vi "e.gate ASCII Write Value - Boolean.vi"(6 "Value":bool, 8 "error in (no error)":errorcluster, 9 "Channel":i32, 11 "e.gate Configuration In":T1) -> (0 "error out":errorcluster, 3 "connection ID Out":T1)   [LabVIEW 2016]
doc: "<B>AMC - Analytik & Messtechnik GmbH Chemnitz</B>\n\nLabVIEW Drivers for e.gate / e.pac series from Gantner Instruments\n\nThis VI writes a value specified by <B>Channel</B> to a device specified by <B>connection ID In</B>."
uses:
  e.gate Configuration.ctl
  e.gate Channel Data.ctl
  e.gate Data Type.ctl
  e.gate Protocol Type.ctl
  e.gate Module  Data.ctl
  e.gateHSP_DLLhandle.ctl
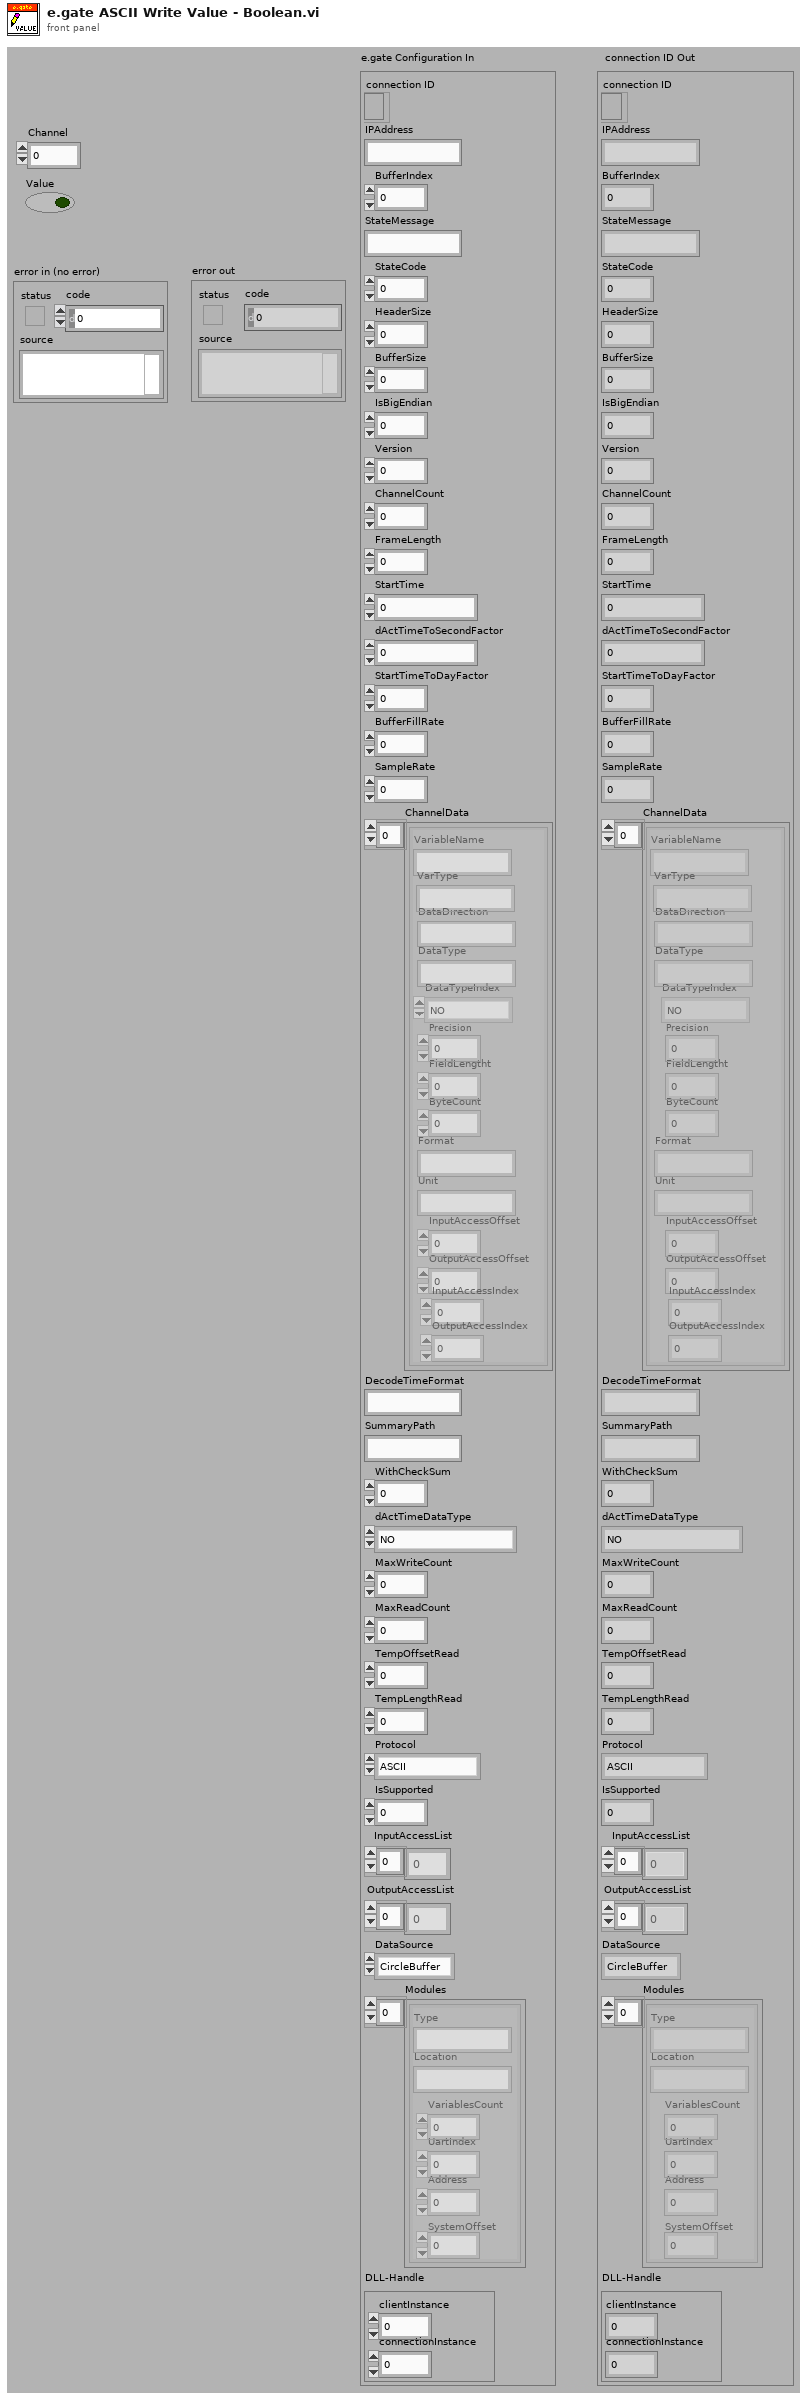
[diagram p1: front panel]
types:
  T1 = typedef "e.gate Configuration.ctl" = cluster{"connection ID":refnum<k5>, "IPAddress":string, "BufferIndex":i32, "StateMessage":string, "StateCode":i8, "HeaderSize":i32, "BufferSize":i32, "IsBigEndian":i32, "Version":i32, "ChannelCount":i32, "FrameLength":i32, "StartTime":dbl, "dActTimeToSecondFactor":dbl, "StartTimeToDayFactor":dbl, "BufferFillRate":dbl, "SampleRate":dbl, "ChannelData":T2[], "DecodeTimeFormat":string, "SummaryPath":string, "WithCheckSum":i32, "dActTimeDataType":T3, "MaxWriteCount":i32, "MaxReadCount":i32, "TempOffsetRead":i32, "TempLengthRead":i32, "Protocol":T4, "IsSupported":i32, "InputAccessList":i32[], "OutputAccessList":i32[], "DataSource":enum16{"CircleBuffer", "test.con Logger", "test.con Archive"}, "Modules":T5[], "DLL-Handle":T6}
  T2 = typedef "e.gate Channel Data.ctl" = cluster{"VariableName":string, "DataDirection":string, "DataType":string, "DataTypeIndex":T3, "Precision":i16, "FieldLengtht":i16, "ByteCount":i32, "Format":string, "Unit":string, "InputAccessOffset":i32, "OutputAccessOffset":i16, "InputAccessIndex":i16, "OutputAccessIndex":i16, "VarType":string}
  T3 = typedef "e.gate Data Type.ctl" = enum16{"NO", "BOOL", "SINT8", "USINT8", "SINT16", "USINT16", "SINT32", "USINT32", "FLOAT", "SET8", "SET16", "SET32", "DOUBLE", "SINT64", "USINT64", "SET64"}
  T4 = typedef "e.gate Protocol Type.ctl" = enum16{"ASCII", "HighspeedPort Online", "HighspeedPort Buffer", "eGateHighspeedPortDLL "}
  T5 = typedef "e.gate Module  Data.ctl" = cluster{"Type":string, "Location":string, "VariablesCount":i16, "UartIndex":i16, "Address":i16, "SystemOffset":i16}
  T6 = typedef "e.gateHSP_DLLhandle.ctl" = cluster{"clientInstance":i32, "connectionInstance":i32}
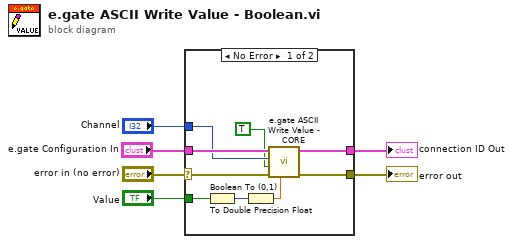
[diagram p0: block diagram]
diagram:
  n1 = case shown="No Error" "error in (no error)" {
    selector: "error in (no error)" -> [w15 w17]
    tunnel: "e.gate Configuration In" -> [w14 w16]
    tunnel: "Channel" -> [w8 _]
    tunnel: [w13 w16] -> w3
    tunnel: [w12 w17] -> w2
    tunnel: "Value" -> [w11 _]
    frame No Error {
      n2 = Boolean To (0,1)(Boolean=w11) -> (0, 1=w9:i16)
      n3 = To Double Precision Float(number=w9) -> (double precision float=w10:dbl)
      n4 = call "e.gate ASCII Write Value - CORE.vi"("Value"=w10, "error in (no error)"=w15, "Boolean"=TRUE, "Channel"=w8, "e.gate Configuration In"=w14) -> ("error out"=w12:errorcluster, "e.gate Configuration Out"=w13:T1)  [unwired: 5 out]
    }
    frame Error {
    }
  }
  "error out" <- w2
  "connection ID Out" <- w3
